vi "ntr.flow-panel.set-ref.vi"(6 "Enum":T1=enum."Out of Range", 8 "String Message":string, 10 "Element Name":string, 11 "refs":refnum<vi>[](array[refnum])) -> (1 "Missing Element? (error)":bool)   [LabVIEW 2024]
uses:
  controls/type.nrt.elment-state.ctl
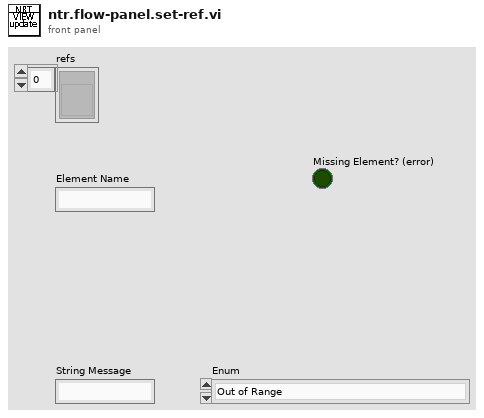
[diagram p1: front panel]
types:
  T1 = typedef "type.nrt.elment-state.ctl" = enum16{"No Change", "OFF", "In Range", "Out of Range", "Alarm"}
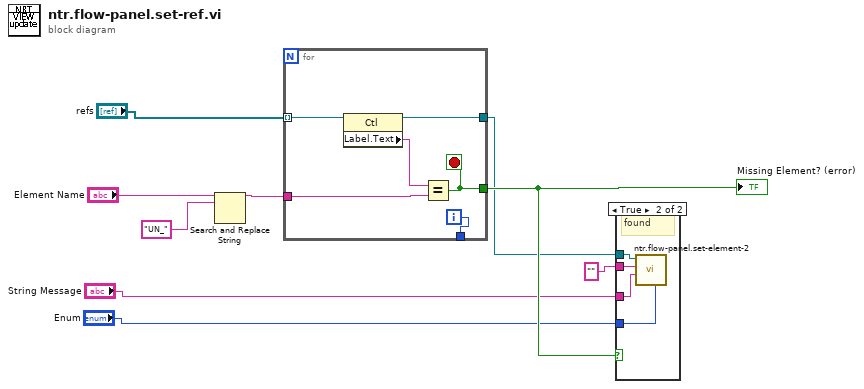
[diagram p0: block diagram]
diagram:
  n1 = Search and Replace String(input string="Element Name", search string="UN_") -> (result string=w1:string)  [unwired: 6 in, 3 out]
  n2 = for {
    tunnel: "refs" -> [w15] mode=indexing
    tunnel: [w14] -> w5
    tunnel: w1 -> [w13]
    tunnel: [w11] -> _
    tunnel: [w10] -> w9
    i -> [w11]
    stop <- w10 stop-if-true
    n3 = property class="Ctl"(reference=w15) -> (reference out=w14:refnum<vi>, "Label.Text"=w12:string)  [unwired: 1 in, 1 out]
    n4 = Equal?(x=w12, y=w13) -> (x = y?=w10:bool)
  }
  "Missing Element? (error)" <- w9
  n5 = case shown="True" w9 {
    tunnel: w5 -> [_ w19]
    tunnel: "" ("Boolean msg (empty: Don't change)") -> [_ w18]
    tunnel: "String Message" -> [_ w17]
    tunnel: "Enum" -> [_ w16]
    frame False {
    }
    frame True {
      # "found"
      n6 = call "ntr.flow-panel.set-element-2.vi"("Enum 2"=w16, "Message Text"=w17, "Boolean Text (empty: no change)"=w18, "Ctl Refnum"=w19) -> ()  [unwired: 7 in, 1 out]
    }
  }
